vi "Robot to Dashboard Comm.vi"   [LabVIEW 2012]
uses:
  Robot Global Data.vi
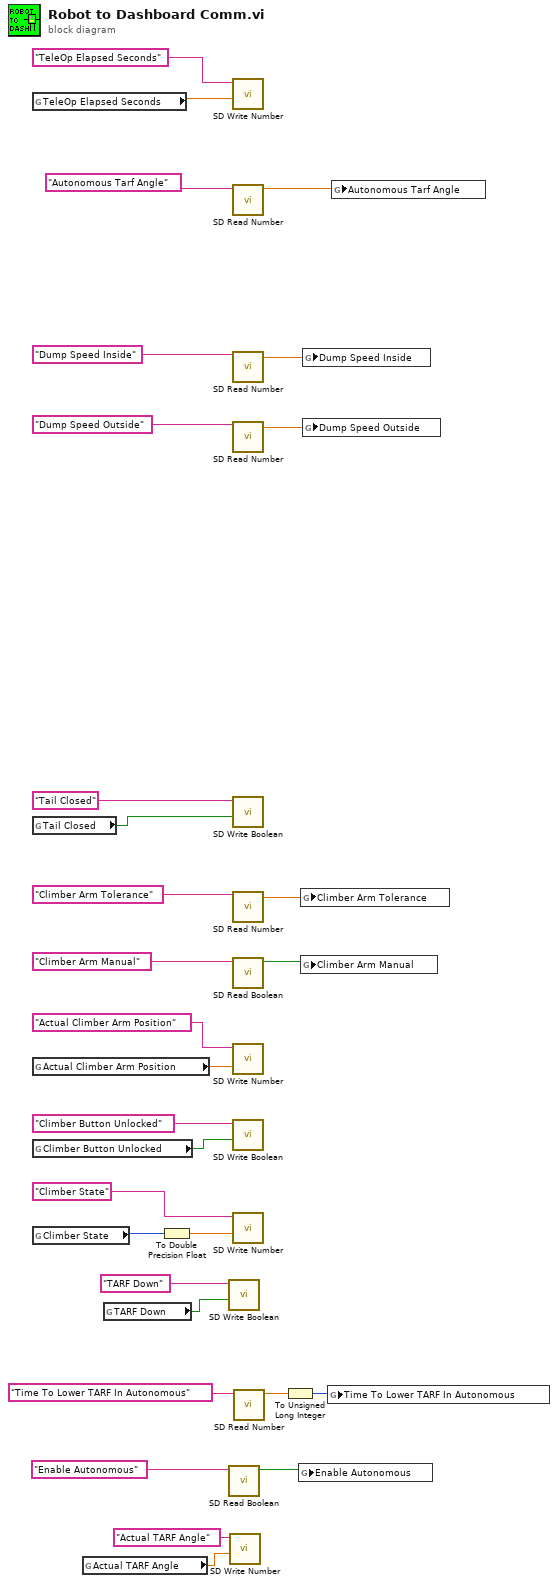
[diagram p0: block diagram]
diagram:
  n1 = global read "Robot Global Data.vi" "TeleOp Elapsed Seconds"() -> (w15:dbl)
  n2 = global read "Robot Global Data.vi" "Tail Closed"() -> (w29:bool)
  n3 = global read "Robot Global Data.vi" "Actual Climber Arm Position"() -> (w19:dbl)
  n4 = global read "Robot Global Data.vi" "Climber Button Unlocked"() -> (w16:bool)
  n5 = global read "Robot Global Data.vi" "Climber State"() -> (w12:u8)
  n6 = global read "Robot Global Data.vi" "Actual TARF Angle"() -> (w1:dbl)
  n7 = global read "Robot Global Data.vi" "TARF Down"() -> (w9:bool)
  n8 = To Double Precision Float(number=w12) -> (double precision float=w13:dbl)
  n9 = call <vilib>:"SD Write Boolean.vi"("Boolean"=w9, "Name"="TARF Down") -> ()  [unwired: 8 in, 2 out]
  n10 = call <vilib>:"SD Read Boolean.vi"("Name"="Enable Autonomous") -> ("Boolean"=w3:bool)  [unwired: 8 in, 2 out]
  n11 = call <vilib>:"SD Write Number.vi"("Numeric"=w1, "Name"="Actual TARF Angle") -> ()  [unwired: 8 in, 2 out]
  n12 = call <vilib>:"SD Write Number.vi"("Numeric"=w15, "Name"="TeleOp Elapsed Seconds") -> ()  [unwired: 8 in, 2 out]
  n13 = call <vilib>:"SD Read Number.vi"("Name"="Autonomous Tarf Angle") -> ("Numeric"=w8:dbl)  [unwired: 8 in, 2 out]
  n14 = call <vilib>:"SD Read Number.vi"("Name"="Dump Speed Inside") -> ("Numeric"=w23:dbl)  [unwired: 8 in, 2 out]
  n15 = call <vilib>:"SD Read Number.vi"("Name"="Dump Speed Outside") -> ("Numeric"=w21:dbl)  [unwired: 8 in, 2 out]
  n16 = call <vilib>:"SD Write Boolean.vi"("Boolean"=w29, "Name"="Tail Closed") -> ()  [unwired: 8 in, 2 out]
  n17 = call <vilib>:"SD Read Number.vi"("Name"="Climber Arm Tolerance") -> ("Numeric"=w28:dbl)  [unwired: 8 in, 2 out]
  n18 = call <vilib>:"SD Read Boolean.vi"("Name"="Climber Arm Manual") -> ("Boolean"=w25:bool)  [unwired: 8 in, 2 out]
  n19 = call <vilib>:"SD Write Number.vi"("Numeric"=w19, "Name"="Actual Climber Arm Position") -> ()  [unwired: 8 in, 2 out]
  n20 = call <vilib>:"SD Write Boolean.vi"("Boolean"=w16, "Name"="Climber Button Unlocked") -> ()  [unwired: 8 in, 2 out]
  n21 = call <vilib>:"SD Write Number.vi"("Numeric"=w13, "Name"="Climber State") -> ()  [unwired: 8 in, 2 out]
  n22 = call <vilib>:"SD Read Number.vi"("Name"="Time To Lower TARF In Autonomous") -> ("Numeric"=w7:dbl)  [unwired: 8 in, 2 out]
  n23 = To Unsigned Long Integer(number=w7) -> (unsigned 32bit integer=w6:u32)
  n24 = global write "Robot Global Data.vi" "Enable Autonomous"(w3) -> ()
  n25 = global write "Robot Global Data.vi" "Climber Arm Tolerance"(w28) -> ()
  n26 = global write "Robot Global Data.vi" "Climber Arm Manual"(w25) -> ()
  n27 = global write "Robot Global Data.vi" "Dump Speed Inside"(w23) -> ()
  n28 = global write "Robot Global Data.vi" "Dump Speed Outside"(w21) -> ()
  n29 = global write "Robot Global Data.vi" "Time To Lower TARF In Autonomous"(w6) -> ()
  n30 = global write "Robot Global Data.vi" "Autonomous Tarf Angle"(w8) -> ()
